vi "Add Sheet.vi"(8 "error in":errorcluster, 10 "Sheet Name":string, 11 "SpreadsheetDoc in":refnum<k24>) -> (0 "error out":errorcluster, 3 "SpreadsheetDoc out":refnum<k24>)   [LabVIEW 2019, in "Open Xml.lvlib"]
uses:
  Open Xml.lvlib
  D:/git/Open-Xml-LabVIEW/Source/DocumentFormat.OpenXml.dll
  DocumentFormat.OpenXml.dll
  D:/git/Open-Xml-LabVIEW/Source/DocumentFormat.OpenXml.Framework.dll
  DocumentFormat.OpenXml.Framework.dll
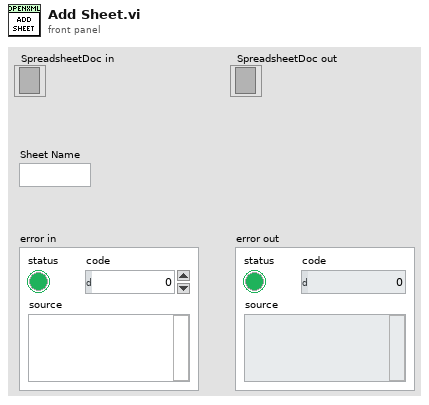
[diagram p1: front panel]
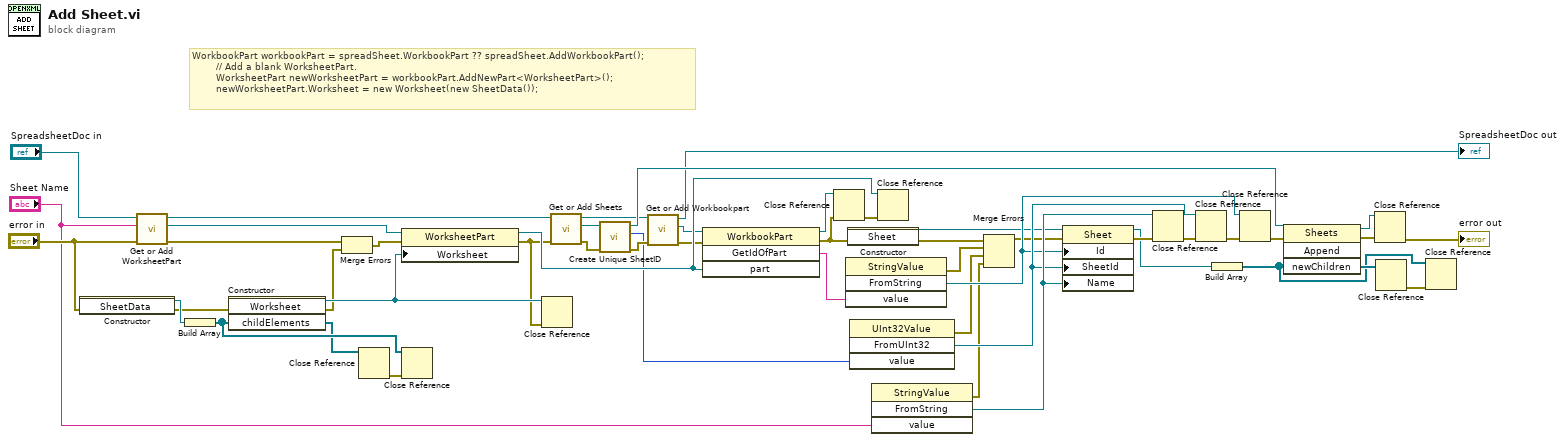
[diagram p0: block diagram]
diagram:
  # "WorkbookPart workbookPart = spreadSheet.WorkbookPart ?? spreadSheet.AddWorkbookPart();\n        // Add a blank WorksheetPart.\n        WorksheetPart newWorksheetPart = workbookPart.AddNewPart<WorksheetPart>();\n        newWorksheetPart.Worksheet = new Worksheet(new SheetData());"
  n1 = constructor class="SheetData"(error in="error in") -> (reference out=w17:refnum<k24>, error out=w16:errorcluster)  [unwired: 2 in, 1 out]
  n2 = call "Get or Add WorksheetPart.vi"("error in"="error in", "Sheet Name"="Sheet Name", "SpreadsheetDoc in"="SpreadsheetDoc in") -> ("error out"=w22:errorcluster, "WorksheetPart"=w18:refnum<k24>, "SpreadsheetDoc out"=w27:refnum<k24>)  [unwired: 6 in]
  n3 = Build Array(w17) -> (w21:refnum<k24>[])
  n4 = constructor class="Worksheet"(error in=w16, "childElements"=w21) -> (reference out=w26:refnum<k24>, error out=w25:errorcluster, "childElements"=w20:refnum<k24>[])  [unwired: 2 in, 1 out]
  n5 = Merge Errors(w22, w25) -> (w24:errorcluster)
  n6 = Close Reference(reference=w20) -> (error out=w19:errorcluster)  [unwired: 1 in]
  n7 = property on="New WorksheetPart" class="WorksheetPart"(reference=w18, error in=w24, "Worksheet"=w26) -> (reference out=w43:refnum<k24>, error out=w8:errorcluster)
  n8 = Close Reference(reference=w21, error in (no error)=w19) -> ()  [unwired: 1 out]
  n9 = Close Reference(reference=w26, error in (no error)=w8) -> ()  [unwired: 1 out]
  n10 = call "Get or Add Sheets.vi"("error in"=w8, "SpreadsheetDoc in"=w27) -> ("error out"=w46:errorcluster, "Sheets"=w44:refnum<k24>, "SpreadsheetDoc out"=w30:refnum<k24>)  [unwired: 7 in]
  n11 = call "Create Unique SheetID.vi"("error in"=w46, "Sheets in"=w44) -> ("error out"=w47:errorcluster, "Unique SheetID"=w33:u32, "Sheets out"=w45:refnum<k24>)  [unwired: 7 in]
  n12 = call "Get or Add Workbookpart.vi"("error in"=w47, "SpreadsheetDoc in"=w30) -> ("error out"=w29:errorcluster, "WorkbookPart"=w28:refnum<k24>, "SpreadsheetDoc out"=→"SpreadsheetDoc out":refnum<k24>)  [unwired: 7 in]
  n13 = invoke class="WorkbookPart" method="GetIdOfPart"(reference=w28, error in=w29, "part"=w43) -> (reference out=w48:refnum<k24>, error out=w6:errorcluster, "GetIdOfPart"=w32:string)  [unwired: 1 in, 1 out]
  n14 = Close Reference(reference=w48, error in (no error)=w6) -> (error out=w7:errorcluster)
  n15 = invoke class="StringValue" method="FromString"("value"=w32) -> (error out=w3:errorcluster, "FromString"=w35:refnum<k24>)  [unwired: 3 in, 2 out]
  n16 = constructor class="Sheet"(error in=w6) -> (reference out=w31:refnum<k24>, error out=w4:errorcluster)  [unwired: 2 in, 1 out]
  n17 = invoke class="UInt32Value" method="FromUInt32"("value"=w33) -> (error out=w2:errorcluster, "FromUInt32"=w37:refnum<k24>)  [unwired: 3 in, 2 out]
  n18 = invoke class="StringValue" method="FromString"("value"="Sheet Name") -> (error out=w10:errorcluster, "FromString"=w38:refnum<k24>)  [unwired: 3 in, 2 out]
  n19 = Close Reference(reference=w43, error in (no error)=w7) -> ()  [unwired: 1 out]
  n20 = Merge Errors(w4, w3, w2, w10) -> (w5:errorcluster)
  n21 = property class="Sheet"(reference=w31, error in=w5, "Id"=w35, "SheetId"=w37, "Name"=w38) -> (reference out=w15:refnum<k24>, error out=w34:errorcluster)
  n22 = Close Reference(reference=w38, error in (no error)=w34) -> (error out=w1:errorcluster)
  n23 = Close Reference(reference=w37, error in (no error)=w1) -> (error out=w36:errorcluster)
  n24 = Build Array(w15) -> (w12:refnum<k24>[])
  n25 = Close Reference(reference=w35, error in (no error)=w36) -> (error out=w39:errorcluster)
  n26 = invoke class="Sheets" method="Append"(reference=w45, error in=w39, "newChildren"=w12) -> (reference out=w40:refnum<k24>, error out=w41:errorcluster, "newChildren"=w14:refnum<k24>[])  [unwired: 1 in, 1 out]
  n27 = Close Reference(reference=w40, error in (no error)=w41) -> (error out=→"error out":errorcluster)
  n28 = Close Reference(reference=w14) -> (error out=w13:errorcluster)  [unwired: 1 in]
  n29 = Close Reference(reference=w12, error in (no error)=w13) -> ()  [unwired: 1 out]
